vi "Act on Action.vi"(8 "error in (no error)":errorcluster, 10 "Project Builder in":refnum<class "Project Builder.lvclass">, 11 "Project Action in":refnum<class "Project Action.lvclass">) -> (0 "error out":errorcluster, 1 "Continue?":bool, 2 "Project Builder out":refnum<class "Project Builder.lvclass">)   [LabVIEW 2019, in "ProjectBuilder.lvlib" / "Project Builder.lvclass"]
doc: "Call 'Act on Action_Do' if not a report action. If report action call 'Report_Do' instead."
uses:
  Project Builder.lvclass
  Project Action/Project Action.lvclass
  Report Action/Report Action/Report Action.lvclass
  ProjectBuilder.lvlib
  Data/Report Data/Report Data.lvclass
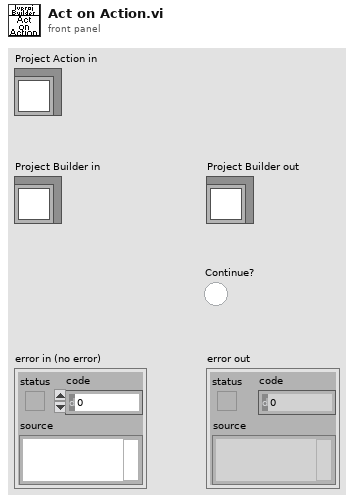
[diagram p1: front panel]
types:
  T1 = typedef "ProjectBuilder.lvlib/Ctl_Build Steps.ctl" = enum16{"Source Test", "Build", "Post-Build Test", "Deploy", "Report"}
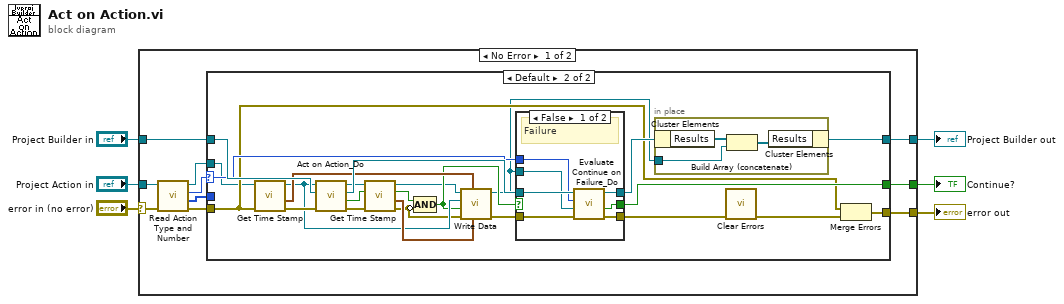
[diagram p0: block diagram]
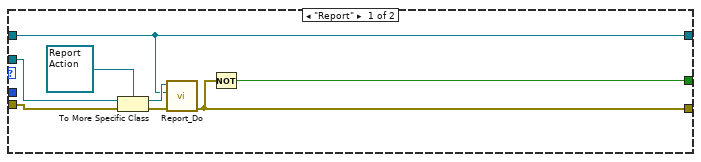
[diagram p2: hidden frame]
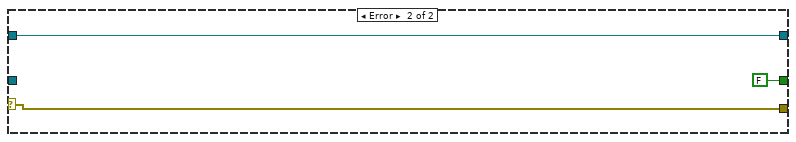
[diagram p4: hidden frame]
diagram:
  n1 = case shown="No Error" "error in (no error)" {
    selector: "error in (no error)" -> [w13 w61]
    tunnel: [w16 w61] -> w5
    tunnel: [w8 w60] -> w3
    tunnel: "Project Builder in" -> [w15 w60]
    tunnel: [w7 FALSE] -> w2
    tunnel: "Project Action in" -> [w14 _]
    frame No Error {
      n2 = call "Read Action Type and Number.vi"("error in (no error)"=w13, "Project Action in"=w14) -> ("error out"=w12:errorcluster, "Action Number"=w10:i32[], "Build Step"=w11:T1, "Project Action out"=w9:refnum<class "Project Action.lvclass">)  [unwired: 6 in]
      n3 = case shown="Default" w11 {
        selector: w11 -> [_ w41]
        tunnel: [w18 w36] -> w16
        tunnel: w15 -> [w19 w45]
        tunnel: w12 -> [w22 w34]
        tunnel: w10 -> [_ _]
        tunnel: w9 -> [w24 w30]
        tunnel: [w19 w44] -> w8
        tunnel: [w17 w40] -> w7
        frame "Report" {
          n4 = To More Specific Class(target class=refnum<class "Report Action.lvclass"> refnum ("Report Action in"), reference=w24, error in=w22) -> (specific class reference=w21:refnum<class "Report Action.lvclass">, error out=w20:errorcluster)
          n5 = call-dynamic "Report_Do.vi"("error in (no error)"=w20, "Project Builder in"=w19, "Report Action in"=w21) -> ("error out"=w18:errorcluster)  [unwired: 8 in]
          n6 = Not(x=w18) -> (.not. x?=w17:bool)
        }
        frame Default {
          n7 = call "Get Time Stamp.vi"("error in (no error)"=w34) -> ("error out"=w35:errorcluster, "Seconds since 1Jan1904"=w32:timestamp)  [unwired: 9 in]
          n8 = call-dynamic "Act on Action_Do.vi"("error in (no error)"=w35, "Project Builder in"=w45, "Project Action in"=w30) -> ("error out"=w33:errorcluster, "Success?"=w39:bool, "Project Builder out"=w43:refnum<class "Project Builder.lvclass">, "Report"=w26:refnum<class "Report Data.lvclass">)  [unwired: 5 in]
          n9 = call "Get Time Stamp.vi"("error in (no error)"=w33) -> ("error out"=w28:errorcluster, "Seconds since 1Jan1904"=w31:timestamp)  [unwired: 9 in]
          n10 = Compound Arithmetic op=AND(w39, invert w28) -> (w29:bool)
          n11 = call "Write Data.vi"("Time End"=w31, "Time Start"=w32, "error in"=w28, "Success?"=w29, "Project Action"=w30, "Report Data in"=w26) -> ("error dub"=w27:errorcluster, "Report Data out"=w25:refnum<class "Report Data.lvclass">)  [unwired: 4 in]
          n12 = case shown="False" w29 {
            selector: w29 -> [_ w53]
            tunnel: w43 -> [w52 w55]
            tunnel: [w51 w55] -> w42
            tunnel: w27 -> [w50 w54]
            tunnel: [w49 w54] -> w38
            tunnel: w41 -> [w48 _]
            tunnel: [w47 w53] -> w40
            tunnel: w25 -> [w46 _]
            frame False {
              # "Failure"
              n13 = call-dynamic "Evaluate Continue on Failure_Do.vi"("error in (no error)"=w50, "Report"=w46, "Build Step"=w48, "Project Builder in"=w52) -> ("error out"=w49:errorcluster, "Continue?"=w47:bool, "Project Builder out"=w51:refnum<class "Project Builder.lvclass">)  [unwired: 5 in]
            }
            frame True {
              # "Success"
            }
          }
          n14 = in-place {
            in-place-border: w25 -> [w57]
            n15 = in-place-cluster #1(w42) -> ("Results"=w58:refnum<class "Report Data.lvclass">[])
            n16 = Build Array (concatenate)(w58, w57) -> (w56:refnum<class "Report Data.lvclass">[])
            n17 = in-place-cluster #1("Results"=w56) -> (w44:refnum<class "Project Builder.lvclass">)
          }
          n18 = call <vilib>:"Clear Errors.vi"("error in (no error)"=w38) -> ("error out"=w37:errorcluster)  [unwired: 5 in, 1 out]
          n19 = Merge Errors(w34, w37) -> (w36:errorcluster)
        }
      }
    }
    frame Error {
    }
  }
  "error out" <- w5
  "Project Builder out" <- w3
  "Continue?" <- w2
